vi "After Launch Init Core.vi"(8 "error in (no error)":errorcluster, 11 "CS++MCS in":refnum<class "CS++MCS.lvclass">) -> (0 "error out":errorcluster, 3 "CS++MCS out":refnum<class "CS++MCS.lvclass">)   [LabVIEW 2016, in "CS++MCS.lvlib" / "CS++MCS.lvclass"]
doc: "Use <b>Pre Launch init.vi</b> method for sanity checks that are supposed to prevent the actor from launching if they fail. Use <B>this</B> method instead to initialize this actor when it has been activated. A corresponding high priority message will become dispatched before the <B>Actor Core.vi</b> is called.\n\n<b>Derived classed should call the parent methode first</b> and their own initialization code after.\n\nRefer also to the ongoing discussion at https://decibel.ni.com/content/message/57394#57394."
uses:
  CS++MCS.lvclass
  CS++MCS.lvclass/CS++MCS.ctl
  CSPP_Core/Actors/CS++DeviceActor/CS++DeviceActor.lvclass
  CSPP_Core/Classes/CS++ProcessVariables/PVConnection/PVConnection.lvclass
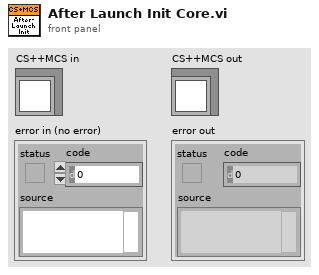
[diagram p1: front panel]
types:
  T1 = cluster{"Read Access":enum8{"Allowed", "Required", "None"}, "Write Access":enum8{"Allowed", "Required", "None"}}
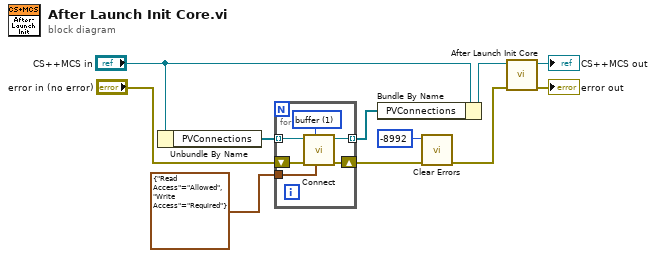
[diagram p0: block diagram]
diagram:
  n1 = Unbundle By Name("CS++MCS in") -> ("PVConnections"=w9:refnum<class "PVConnection.lvclass">[])
  n2 = for {
    tunnel: w9 -> [w17] mode=indexing
    shift-right: [w15] -> w7
    shift-left: "error in (no error)" -> [w16]
    tunnel: [w14] -> w4 mode=indexing
    tunnel: T1 {"Read Access"=enum."Allowed", "Write Access"=enum."Required"} ("Access (R/W allowed)") -> [w13]
    w12 = u16 1 items=["commit", "buffer"] ("Mode (commit)")
    n3 = call "Connect.vi"("Access (R/W allowed)"=w13, "Mode (buffer)"=w12, "Error In"=w16, "PVConnection in"=w17) -> ("Error Out"=w15:errorcluster, "PVConnection out"=w14:refnum<class "PVConnection.lvclass">)  [unwired: 6 in]
  }
  n4 = Bundle By Name(cluster="CS++MCS in", "PVConnections"=w4) -> (w5:refnum<class "CS++MCS.lvclass">)
  n5 = call <vilib>:"Clear Errors.vi"("error in (no error)"=w7, "specific error code to clear (0: all)"=-8992) -> ("error out"=w2:errorcluster)  [unwired: 4 in, 1 out]
  n6 = call-parent "After Launch Init Core.vi"("error in (no error)"=w2, "CS++DeviceActor in"=w5) -> ("error out"=→"error out":errorcluster, "CS++DeviceActor out"=→"CS++MCS out":refnum<class "CS++MCS.lvclass">)  [unwired: 8 in]
